vi "Do.vi"(8 "error in (no error)":errorcluster, 9 "CommandQueueIn":refnum<queue>, 10 "DataNotifierIn":refnum<notifier>, 11 "CommandCopy in":refnum<class "CommandCopy.lvclass">) -> (0 "error out":errorcluster, 1 "ExitFlag":bool, 2 "DataNotifierOut":refnum<notifier>, 3 "CommandCopy out":refnum<class "CommandCopy.lvclass">)   [LabVIEW 2013, in "CommandCopy.lvclass"]
uses:
  CommandCopy.lvclass
  SystemData.lvclass/SystemData.lvclass
  RootCommand.lvclass/RootCommand.lvclass
  SystemData.lvclass/SystemData.lvclass/SystemData.ctl
  Generator.lvclass/Generator.lvclass
panel:
  # "notifier包裝SystemData物件的參考"
  # "命令物件序列參考"
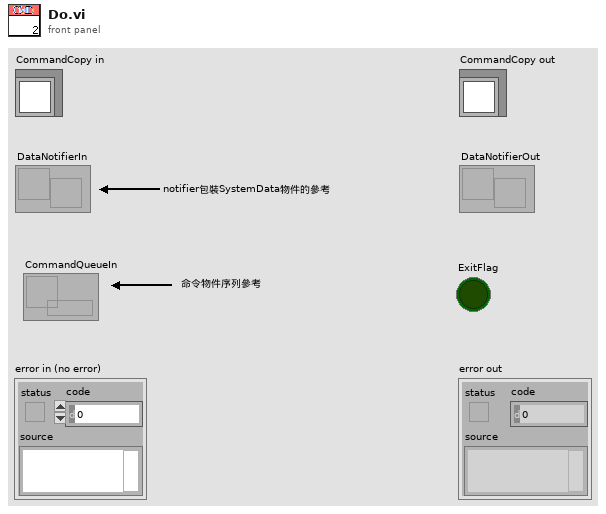
[diagram p1: front panel]
types:
  T1 = typedef "SystemData.lvclass/SystemDataTypeDefine.ctl" = cluster{"ThisVIParameter":cluster{"ThisVIPath":path, "ThisVIReference":refnum<vi>, "AllControlReference":refnum<vi>[]}, "GeneratorParameter":cluster{"Frequency":dbl, "Amplitude":dbl}, "WaveformBuffer":waveform(dbl), "SourceSelect":u16, "GeneratorClassArray":refnum<class "Generator.lvclass">[]}
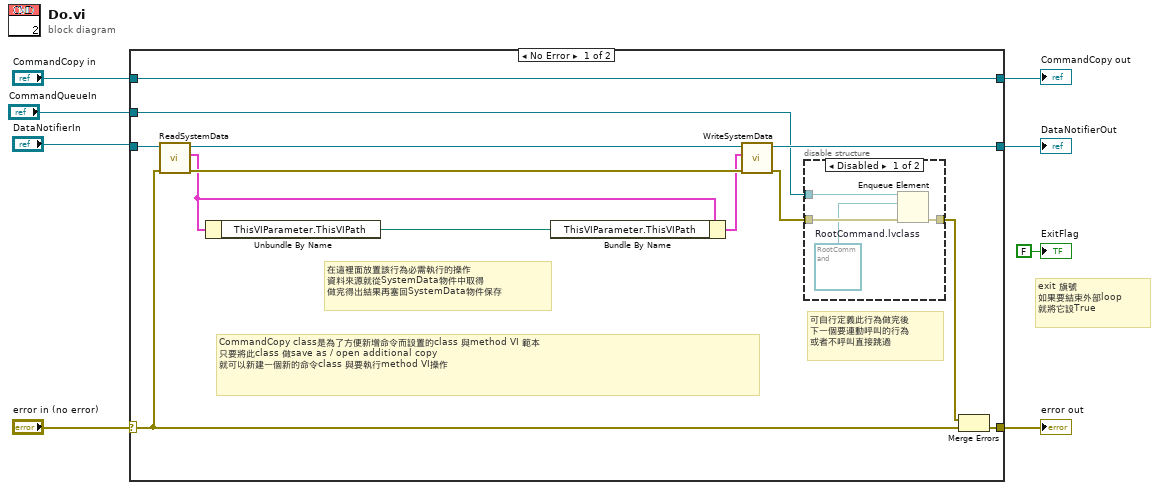
[diagram p0: block diagram]
diagram:
  # "exit 旗號\n如果要結束外部loop\n就將它設True"
  n1 = case shown="No Error" "error in (no error)" {
    selector: "error in (no error)" -> [w10 w29]
    tunnel: [w12 w29] -> w4
    tunnel: [w21 w28] -> w3
    tunnel: "CommandCopy in" -> [w21 w28]
    tunnel: "DataNotifierIn" -> [w20 w27]
    tunnel: [w15 w27] -> w2
    tunnel: "CommandQueueIn" -> [w14 _]
    frame No Error {
      # "CommandCopy class是為了方便新增命令而設置的class 與method VI 範本\n只要將此class 做save as / open additional copy \n就可以新建一個新的命令class 與要執行method VI操作"
      # "在這裡面放置該行為必需執行的操作\n資料來源就從SystemData物件中取得\n做完得出結果再塞回SystemData物件保存"
      # "可自行定義此行為做完後\n下一個要連動呼叫的行為\n或者不呼叫直接跳過"
      n2 = call "ReadSystemData.vi"("error in (no error)"=w10, "DataNotifierIn"=w20) -> ("error out"=w18:errorcluster, "SystemData"=w17:T1, "DataNotifierIn"=w19:refnum<notifier>)  [unwired: 7 in]
      n3 = Unbundle By Name(w17) -> ("ThisVIParameter.ThisVIPath"=w9:path)
      n4 = Bundle By Name(cluster=w17, "ThisVIParameter.ThisVIPath"=w9) -> (w16:T1)
      n5 = call "WriteSystemData.vi"("error in (no error)"=w18, "SystemData"=w16, "DataNotifierIn"=w19) -> ("error out"=w13:errorcluster, "DataNotifierOut"=w15:refnum<notifier>)  [unwired: 7 in]
      n6 = disable-structure shown="Disabled" {
        disable-tunnel: w14 -> [w25 _]
        disable-tunnel: w13 -> [w24 w26]
        disable-tunnel: [w23 w26] -> w11
        frame Disabled {
          w22 = refnum<class "RootCommand.lvclass"> refnum  # RootCommand.lvclass
          n7 = Enqueue Element(queue=w25, element=w22, error in (no error)=w24) -> (error out=w23:errorcluster)  [unwired: 1 in, 2 out]
        }
        frame Enabled {
        }
      }
      n8 = Merge Errors(w11, w10) -> (w12:errorcluster)
    }
    frame Error {
    }
  }
  "error out" <- w4
  "CommandCopy out" <- w3
  "DataNotifierOut" <- w2
  "ExitFlag" <- FALSE ("ExitFlag")
